vi "HI.vi"() -> ()   [LabVIEW 2012]
uses:
  Conveyer Belt/Conveyer Belt Global Data.vi
  Drive/Drive Global Data.vi
panel:
  in  "Wanted Dead Band Value":dbl
  in  "Slow Speed":dbl
  in  "Mid Speed":dbl
  in  "Fast Speed":dbl
  # "Conveyer Belt"
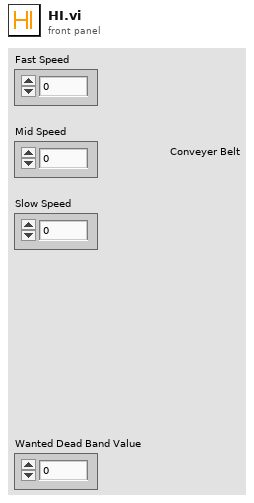
[diagram p1: front panel]
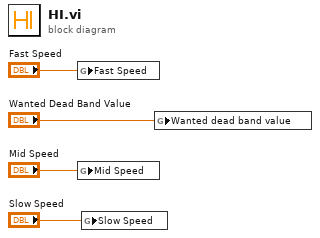
[diagram p0: block diagram]
diagram:
  n1 = global write "Conveyer Belt Global Data.vi" "Fast Speed"("Fast Speed") -> ()
  n2 = global write "Conveyer Belt Global Data.vi" "Mid Speed"("Mid Speed") -> ()
  n3 = global write "Conveyer Belt Global Data.vi" "Slow Speed"("Slow Speed") -> ()
  n4 = global write "Drive Global Data.vi" "Wanted dead band value"("Wanted Dead Band Value") -> ()
